vi "Configure Displayed Units.vi"(7 "Unit Address (1)":u8=1, 8 "error in (no error)":errorcluster, 10 "Displayed Units (0: Degrees C)":u8(ring) items=[" Degrees C", " Degrees F", " Degrees K"], 11 "VISA resource name":refnum<visa-resource-name>) -> (0 "error out":errorcluster, 3 "VISA resource name out":refnum<visa-resource-name>)   [LabVIEW 2014, in "Eurotherm 35xx Series.lvlib"]
doc: "This VI configured temperature units of the instrument. \nChanging this will cause all temperature type parameters to be re-scaled into the new units."
uses:
  <instrlib>/Eurotherm 35xx Series/Eurotherm 35xx Series.lvlib
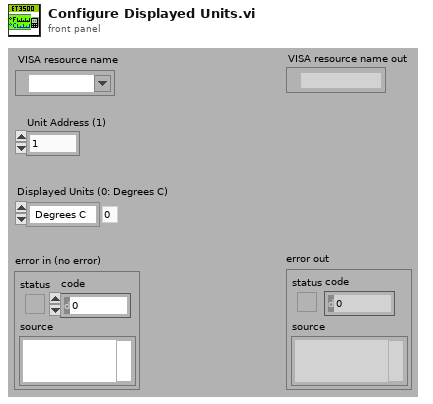
[diagram p1: front panel]
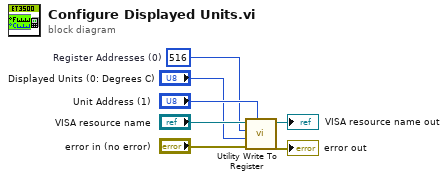
[diagram p0: block diagram]
diagram:
  w1 = 516  # Register Addresses (0)
  n1 = call <instrlib>:"Utility Write To Register.vi"("Unit Address (1)"="Unit Address (1)", "error in (no error)"="error in (no error)", "Data (0)"="Displayed Units (0: Degrees C)", "Register Address (0)"=w1, "VISA resource name"="VISA resource name") -> ("error out"=→"error out":errorcluster, "VISA resource name out"=→"VISA resource name out":refnum<visa-resource-name>)  [unwired: 5 in]
